vi "Send.vi"(10 "Queue Actor":refnum<class "Queue Actor.lvclass">) -> (3 "Last Ack Msg out":refnum<class "Last Ack Msg.lvclass">)   [LabVIEW 2021, in "Last Ack.lvlib" / "Last Ack Msg.lvclass"]
uses:
  Last Ack Msg.lvclass
  Queue Actor/Queue Actor.lvclass
  Last Ack Msg.lvclass/Last Ack Msg.ctl
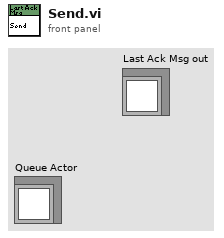
[diagram p1: front panel]
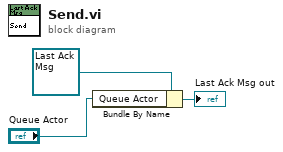
[diagram p0: block diagram]
diagram:
  n1 = Bundle By Name(cluster=refnum<class "Last Ack Msg.lvclass"> refnum ("Last Ack Msg in"), "Queue Actor"="Queue Actor") -> (→"Last Ack Msg out":refnum<class "Last Ack Msg.lvclass">)
